vi "ImageDisplay.vi"(0 "File Path":path=path "C:/Temp/DECODE/14082010501063-Blemish_14_15_42.bmp") -> ()   [LabVIEW 2014]
panel:
  in  "PRESS THE STOP BUTTON TO CONTINUE":bool
  out "new picture":picture
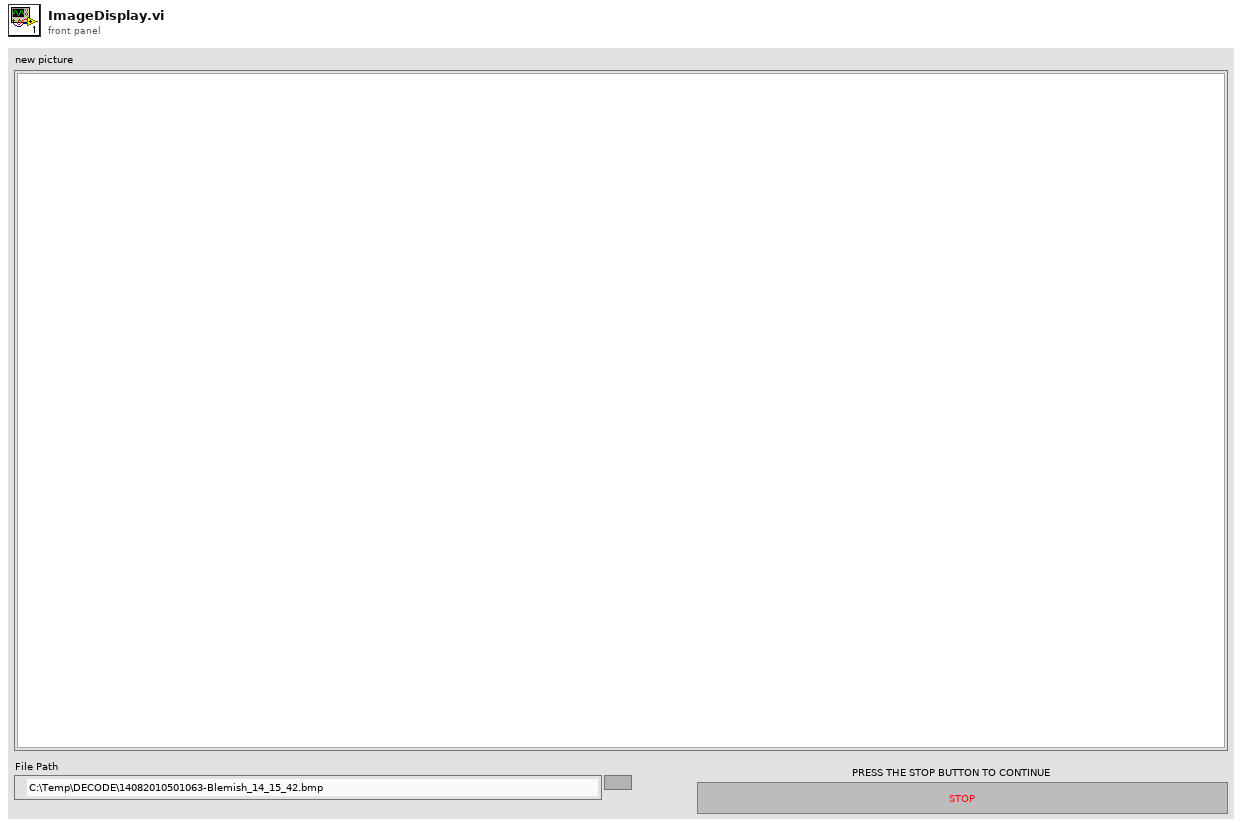
[diagram p1: front panel]
types:
  T1 = typedef "imagedata.ctl" = cluster{"image type":i32, "image depth":i32, "image":u8[], "mask":u8[], "colors":u32[], "Rectangle":cluster{"left":i16, "top":i16, "right":i16, "bottom":i16}}
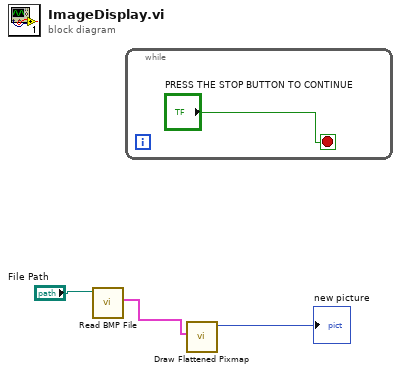
[diagram p0: block diagram]
diagram:
  n1 = call <vilib>:"Read BMP File.vi"("path to BMP file"="File Path") -> ("image data"=w2:T1)  [unwired: 8 in, 2 out]
  n2 = while {
    stop <- "PRESS THE STOP BUTTON TO CONTINUE" stop-if-true
  }
  n3 = call <vilib>:"Draw Flattened Pixmap.vi"("image data"=w2) -> ("new picture"=→"new picture":picture)  [unwired: 8 in]
